vi "Build Search Content For Member.vi"(8 "ItemContent":string, 9 "ItemHeader":string, 10 "Source":string) -> (3 "Result":string)   [LabVIEW 2015, in "UserManagement.lvlib" / "UserBasicInfo.lvclass"]
uses:
  UserManagement/UserBasicInfo/UserBasicInfo.lvclass
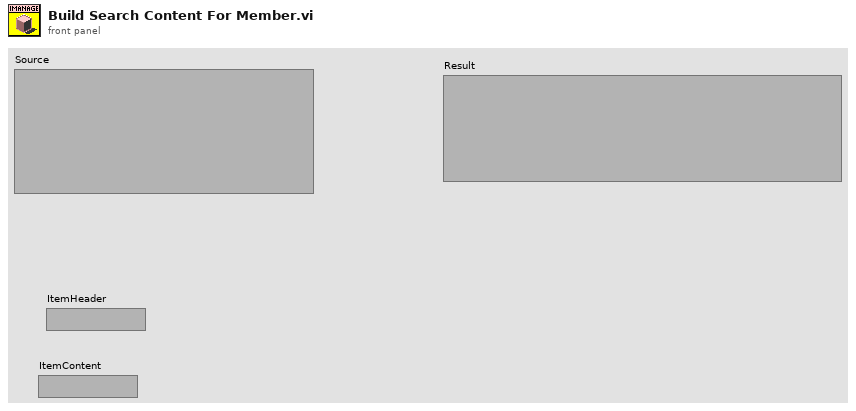
[diagram p1: front panel]
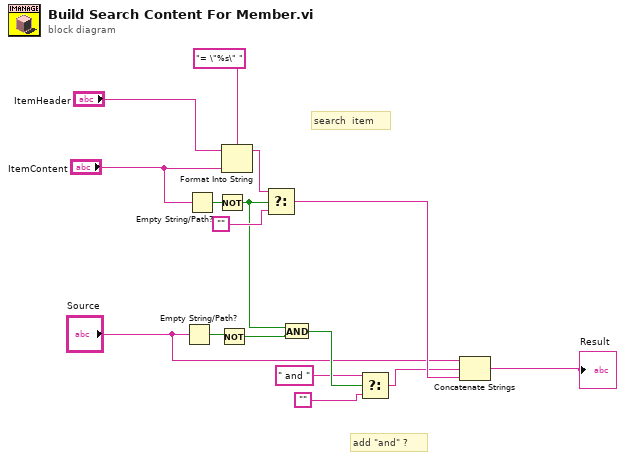
[diagram p0: block diagram]
diagram:
  # "add \"and\" ?"
  # "search  item"
  n1 = Empty String/Path?(string/path="Source") -> (empty?=w9:bool)
  n2 = Empty String/Path?(string/path="ItemContent") -> (empty?=w15:bool)
  n3 = Not(x=w15) -> (.not. x?=w10:bool)
  n4 = Not(x=w9) -> (.not. x?=w8:bool)
  n5 = Format Into String(format string="= \"%s\" ", initial string="ItemHeader", "ItemContent") -> (resulting string=w14:string)  [unwired: 1 in, 1 out]
  n6 = Select(t=w14, s=w10, f="") -> (s? t:f=w7:string)
  n7 = And(x=w10, y=w8) -> (x .and. y?=w5:bool)
  n8 = Select(t=" and ", s=w5, f="") -> (s? t:f=w1:string)
  n9 = Concatenate Strings("Source", w1, w7) -> (→"Result":string)
